vi "Save Failed images.vi"(8 "error in":errorcluster, 9 "Failed Image path":path, 10 "Image Info":T2) -> (0 "error out":errorcluster)   [LabVIEW 2019, in "DataLogger.lvclass"]
doc: "Save Failed Images"
uses:
  DataLogger.lvclass
  <vilib>/vision/Image Controls.llb/IMAQ Image.ctl
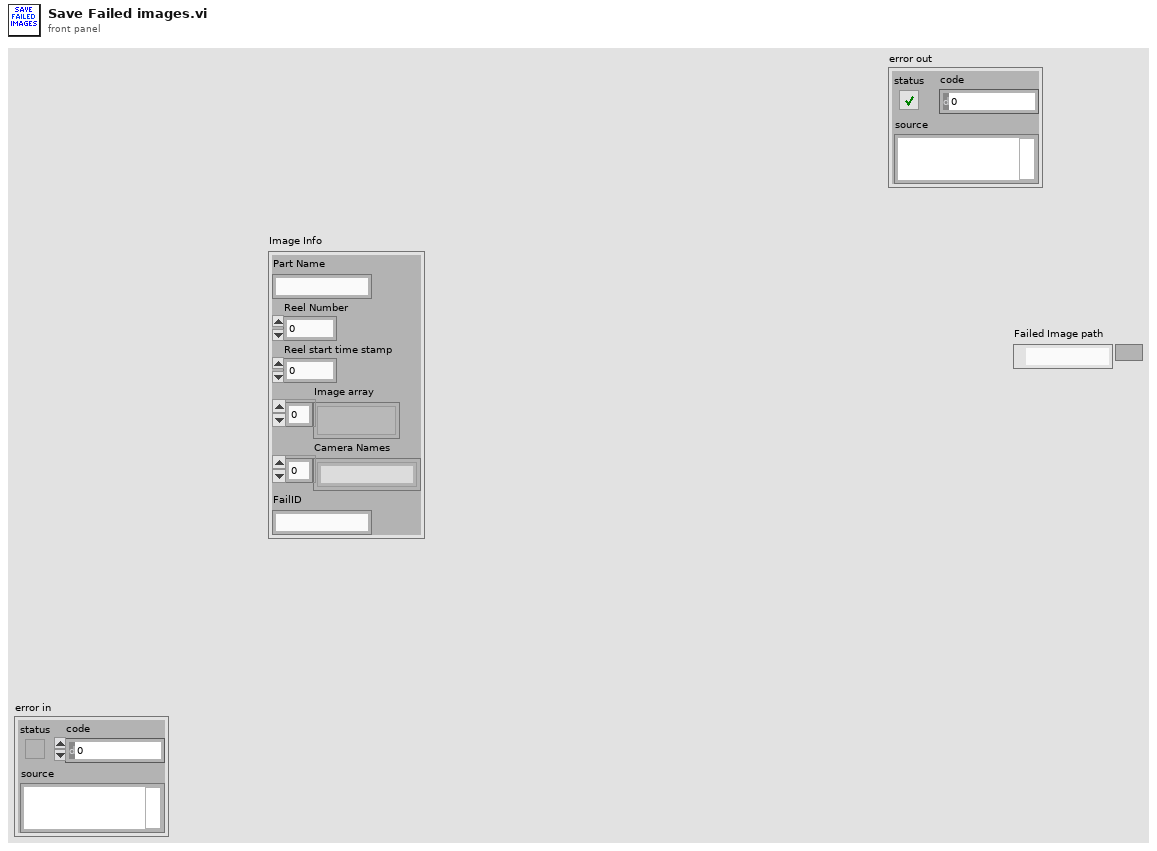
[diagram p1: front panel]
types:
  T1 = typedef "IMAQ Image.ctl" = refnum<image>
  T2 = cluster{"Part Name":string, "Reel Number":u64, "Reel start time stamp":u64, "Image array":T1[], "Camera Names":string[], "FailID":string}
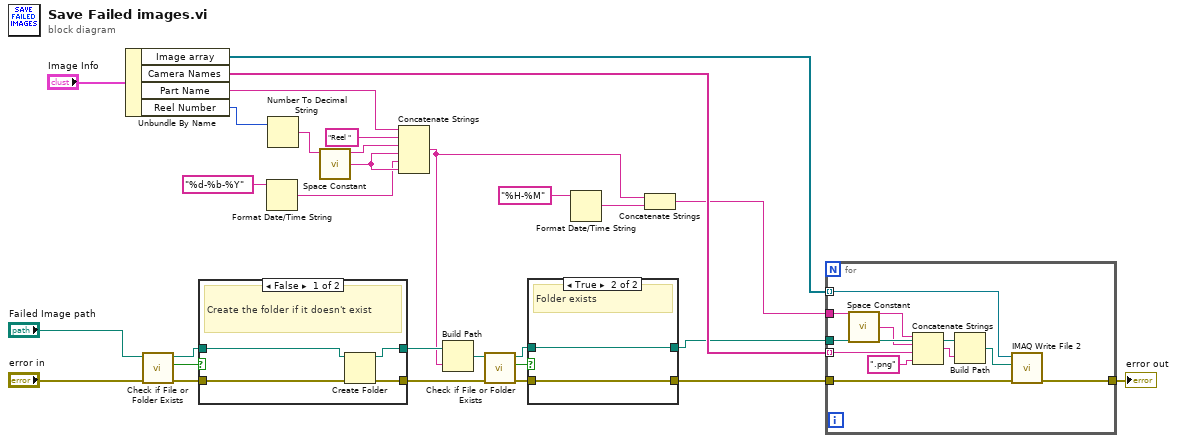
[diagram p0: block diagram]
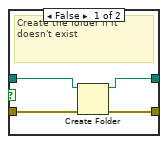
[diagram p2: hidden frame]
diagram:
  n1 = Unbundle By Name("Image Info") -> ("Image array"=w13:T1[], "Camera Names"=w14:string[], "Part Name"=w20:string, "Reel Number"=w19:u64)
  n2 = call <vilib>:"Check if File or Folder Exists.vi"("error in (no error)"="error in", "path"="Failed Image path") -> ("error out"=w23:errorcluster, "file or folder exists?"=w22:bool, "dup path"=w24:path)  [unwired: 7 in]
  n3 = case shown="False" w22 {
    tunnel: w24 -> [w32 w33]
    tunnel: w23 -> [w31 w34]
    tunnel: [w30 w34] -> w17
    tunnel: [w29 w33] -> w21
    frame False {
      # "Create the folder if it doesn't exist"
      n4 = Create Folder(path (use dialog)=w32, error in=w31) -> (created path=w29:path, error out=w30:errorcluster)  [unwired: 1 in, 1 out]
    }
    frame True {
      # "Folder exists"
    }
  }
  n5 = Format Date/Time String(time format string (%c)="%d-%b-%Y") -> (date/time string=w5:string)  [unwired: 2 in]
  n6 = Number To Decimal String(number=w19) -> (decimal integer string=w8:string)  [unwired: 1 in]
  n7 = call <vilib>:"Space Constant.vi"() -> ("String"=w6:string)
  n8 = Concatenate Strings(w20, "Reel " ("string"), w8, w6, w5, w6) -> (w3:string)
  n9 = Build Path(base path=w21, name or relative path=w3) -> (appended path=w18:path)
  n10 = call <vilib>:"Check if File or Folder Exists.vi"("error in (no error)"=w17, "path"=w18) -> ("error out"=w16:errorcluster, "file or folder exists?"=w10:bool, "dup path"=w15:path)  [unwired: 7 in]
  n11 = case shown="True" w10 {
    tunnel: w15 -> [w38 w39]
    tunnel: w16 -> [w37 w40]
    tunnel: [w36 w40] -> w11
    tunnel: [w35 w39] -> w12
    frame False {
      # "Create the folder if it doesn't exist"
      n12 = Create Folder(path (use dialog)=w38, error in=w37) -> (created path=w35:path, error out=w36:errorcluster)  [unwired: 1 in, 1 out]
    }
    frame True {
      # "Folder exists"
    }
  }
  n13 = Format Date/Time String(time format string (%c)="%H-%M") -> (date/time string=w2:string)  [unwired: 2 in]
  n14 = Concatenate Strings(w3, w2) -> (w1:string)
  n15 = for {
    tunnel: w14 -> [w45] mode=indexing
    tunnel: w13 -> [w50] mode=indexing
    tunnel: w12 -> [w48]
    tunnel: w11 -> [w47]
    tunnel: [w46] -> w27
    tunnel: w1 -> [w41]
    n16 = call <vilib>:"Space Constant.vi"() -> ("String"=w42:string)
    n17 = Concatenate Strings(w41, w42, w45, ".png" ("string")) -> (w43:string)
    n18 = Build Path(base path=w48, name or relative path=w43) -> (appended path=w49:path)
    n19 = call-poly "IMAQ Write File 2"("error in (no error)"=w47, "File Path"=w49, "Image"=w50) -> ("error out"=w46:errorcluster)  [unwired: 7 in, 1 out]
  }
  "error out" <- w27
